vi "HW3_2017_WMA.vi"() -> ()   [LabVIEW 2017]
panel:
  in  "OK Button 2":bool
  in  "Path":path
  in  "min":dbl
  in  "hour":dbl
  in  "OK Button":bool
  out "Boolean":bool
  in  "SET ALARM":bool
  out "ALARMING TIME":string
  out "DATE":string
  in  "reinstate":bool
  in  "sec":dbl
  in  "min":dbl
  in  "hour":dbl
  in  "reset":bool
  out "sec":dbl(knob) scale=0.0..60.0
  out "min":dbl(knob) scale=0.0..60.0
  out "hour":dbl(knob) scale=0.0..12.0
  in  "stop":bool
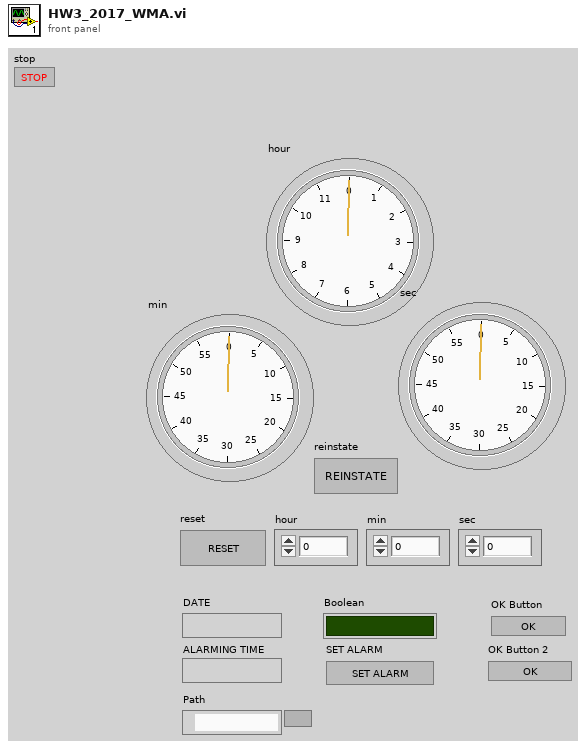
[diagram p1: front panel]
types:
  T1 = typedef "LVDateTimeRec.ctl" = cluster{"fractional second":dbl, "second":i32, "minute":i32, "hour":i32, "day of month":i32, "month":i32, "year":i32, "day of week":i32, "day of year":i32, "DST":i32}
  T2 = typedef "Sound Output Task ID.ctl" = u32
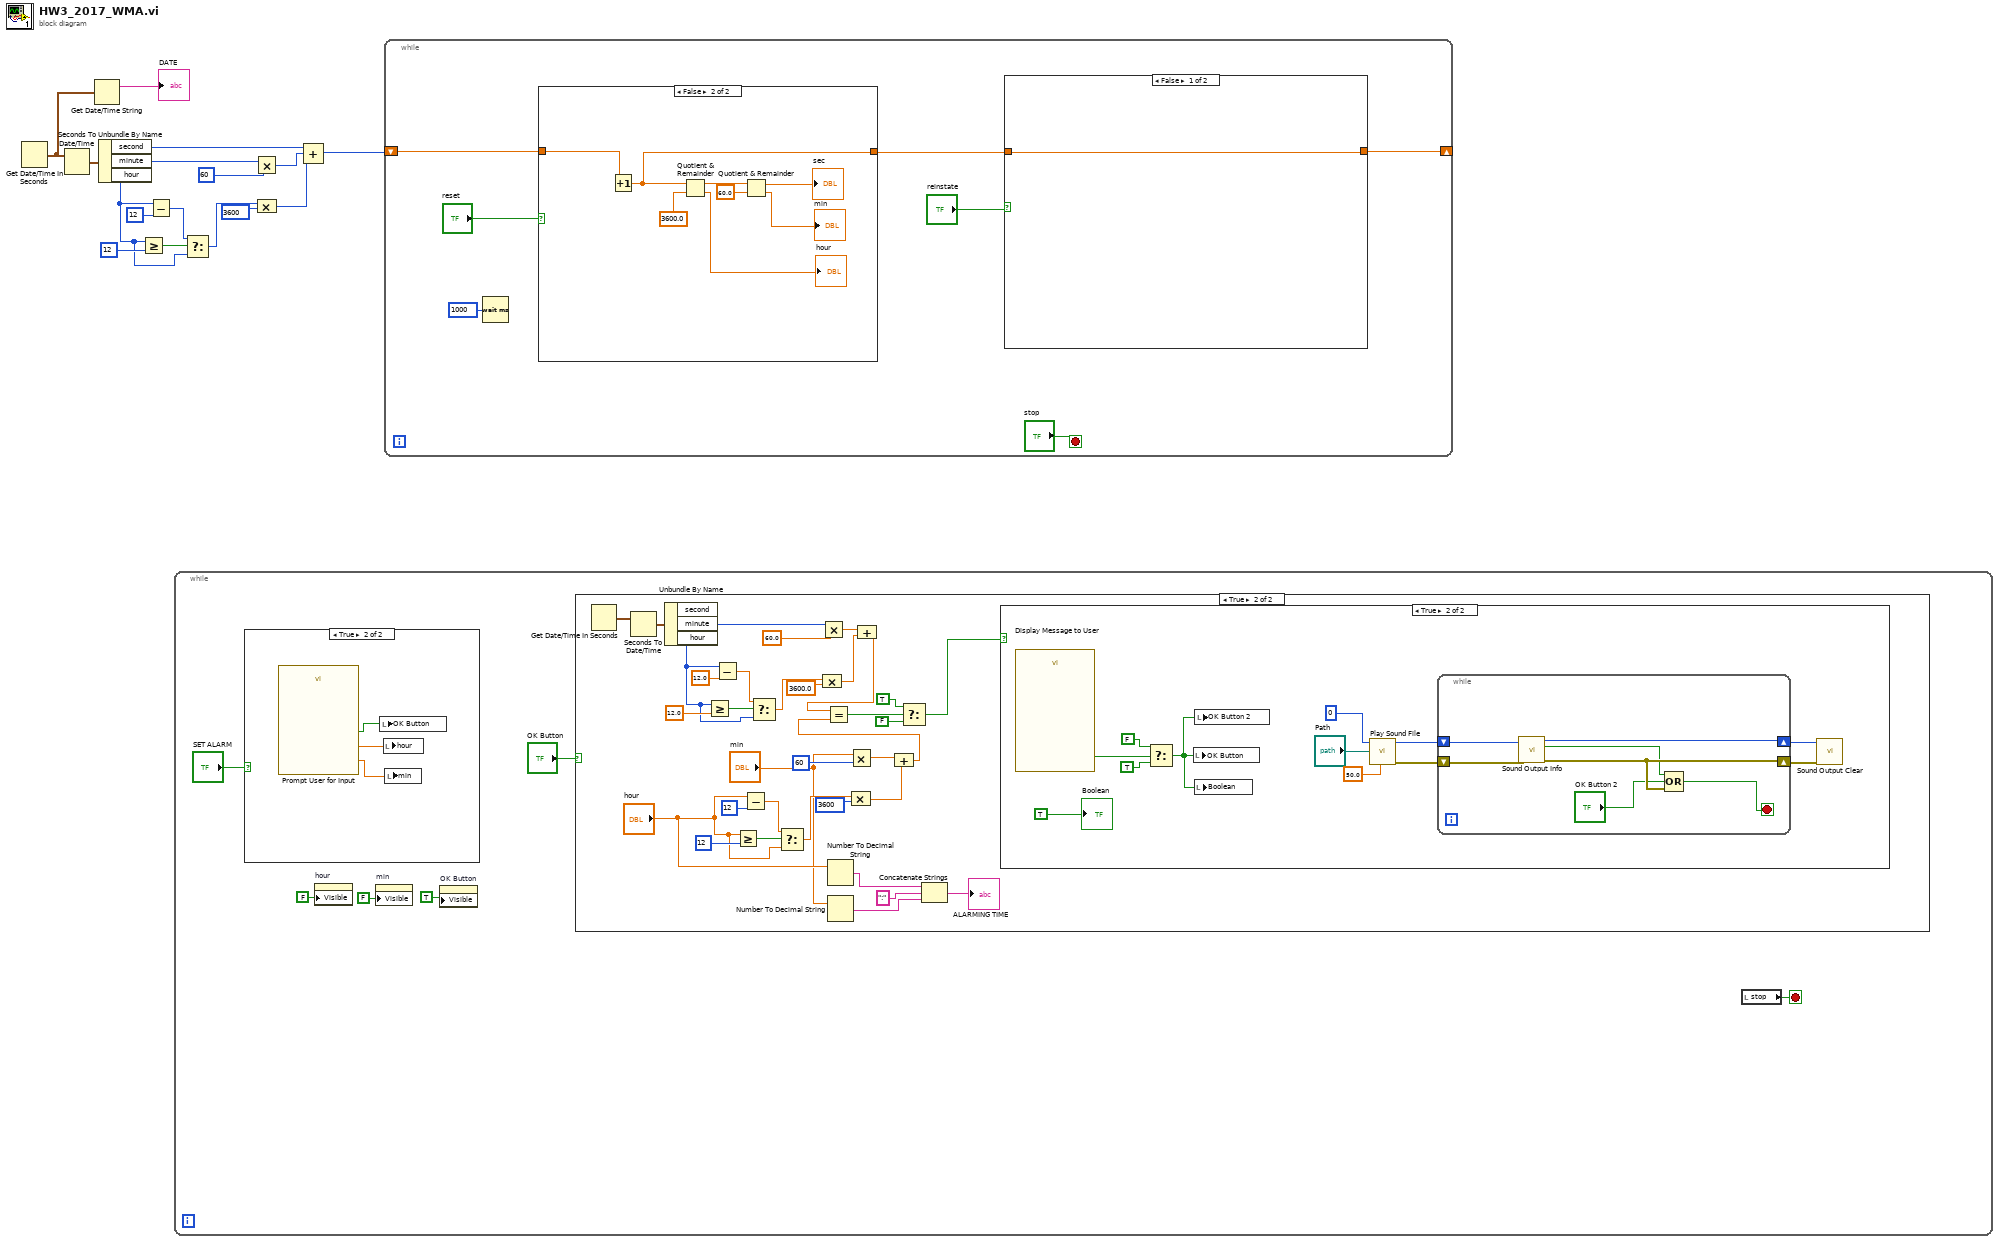
[diagram p0: block diagram]
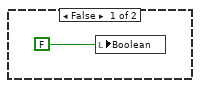
[diagram p3: hidden frame]
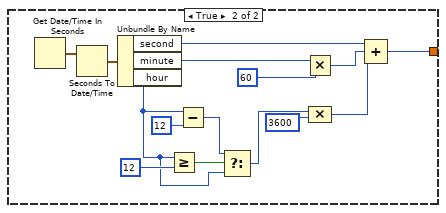
[diagram p5: hidden frame]
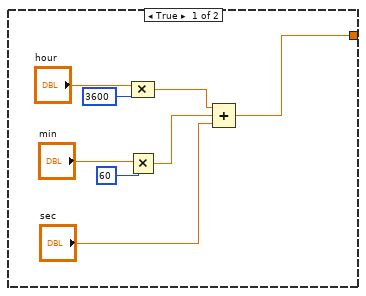
[diagram p6: hidden frame]
diagram:
  n1 = Get Date/Time In Seconds() -> (seconds since 1Jan1904=w5:timestamp)
  n2 = Seconds To Date/Time(time stamp (now)=w5) -> (date time rec=w14:T1)  [unwired: 1 in]
  n3 = Get Date/Time String(seconds (now)=w5) -> (date string=→"DATE":string)  [unwired: 2 in, 1 out]
  n4 = Unbundle By Name(w14) -> ("second"=w12:i32, "minute"=w13:i32, "hour"=w7:i32)
  n5 = Greater Or Equal?(x=w7, y=12) -> (x >= y?=w10:bool)
  n6 = Subtract(x=w7, y=12) -> (x-y=w8:i32)
  n7 = while {
    stop <- w18 stop-if-true
    n8 = case shown="True" "SET ALARM" {
      frame False {
      }
      frame True {
        n9 = call "Prompt User for Input"() -> ("Minute"=w79:dbl, "Hour"=w78:dbl, "OK"=w77:bool)  [unwired: 16 in, 1 out]
        n10 = local write "OK Button"(w77) -> ()
        n11 = local write "hour"(w78) -> ()
        n12 = local write "min"(w79) -> ()
      }
    }
    n13 = property on="hour" class="DigNum (strict)"("Visible"=FALSE) -> ()  [unwired: 2 in, 2 out]
    n14 = property on="min" class="DigNum (strict)"("Visible"=FALSE) -> ()  [unwired: 2 in, 2 out]
    n15 = property on="OK Button" class="Bool (strict)"("Visible"=TRUE) -> ()  [unwired: 2 in, 2 out]
    n16 = case shown="True" "OK Button" {
      frame False {
      }
      frame True {
        n17 = Get Date/Time In Seconds() -> (seconds since 1Jan1904=w26:timestamp)
        n18 = Seconds To Date/Time(time stamp (now)=w26) -> (date time rec=w29:T1)  [unwired: 1 in]
        n19 = Unbundle By Name(w29) -> ("minute"=w30:i32, "hour"=w24:i32)  [unwired: 1 out]
        n20 = Greater Or Equal?(x=w24, y=12.0) -> (x >= y?=w32:bool)
        n21 = Subtract(x=w24, y=12.0) -> (x-y=w34:dbl)
        n22 = Greater Or Equal?(x="hour", y=12) -> (x >= y?=w51:bool)
        n23 = Subtract(x="hour", y=12) -> (x-y=w49:dbl)
        n24 = Select(t=w34, s=w32, f=w24) -> (s? t:f=w35:dbl)
        n25 = Select(t=w49, s=w51, f="hour") -> (s? t:f=w48:dbl)
        n26 = Multiply(x=w30, y=60.0) -> (x*y=w36:dbl)
        n27 = Compound Arithmetic op=MULTIPLY(w35, 3600.0) -> (w37:dbl)
        n28 = Number To Decimal String(number="hour") -> (decimal integer string=w43:string)  [unwired: 1 in]
        n29 = Number To Decimal String(number="min") -> (decimal integer string=w41:string)  [unwired: 1 in]
        n30 = Multiply(x="min", y=60) -> (x*y=w54:dbl)
        n31 = Compound Arithmetic op=MULTIPLY(w48, 3600) -> (w53:dbl)
        n32 = Compound Arithmetic op=ADD(w36, w37) -> (w25:dbl)
        n33 = Compound Arithmetic op=ADD(w54, w53) -> (w47:dbl)
        n34 = Equal?(x=w25, y=w47) -> (x = y?=w46:bool)
        n35 = Select(t=TRUE, s=w46, f=FALSE) -> (s? t:f=w23:bool)
        n36 = Concatenate Strings(w43, ":", w41) -> (→"ALARMING TIME":string)
        n37 = case shown="True" w23 {
          frame False {
            n38 = local write "Boolean"(FALSE ("Boolean")) -> ()
          }
          frame True {
            n39 = call "Display Message to User"() -> ("OK"=w67:bool)  [unwired: 10 in, 1 out]
            n40 = Select(t=FALSE ("Boolean"), s=w67, f=TRUE) -> (s? t:f=w58:bool)
            n41 = local write "OK Button"(w58) -> ()
            n42 = local write "Boolean"(w58) -> ()
            n43 = local write "OK Button 2"(w58) -> ()
            n44 = call <vilib>:"Play Sound File.vi"("timeout (sec)"=50.0, "path"="Path", "device ID"=u32 0) -> ("error out"=w62:errorcluster, "task ID"=w63:T2)  [unwired: 7 in]
            n45 = while {
              shift-right: [w74] -> w61
              shift-left: w63 -> [w76]
              shift-right: [w73] -> w60
              shift-left: w62 -> [w75]
              stop <- w70 stop-if-true
              n46 = call <vilib>:"Sound Output Info.vi"("error in (no error)"=w75, "task ID"=w76) -> ("error out"=w73:errorcluster, "is playing?"=w71:bool, "task ID out"=w74:T2)  [unwired: 6 in, 1 out]
              n47 = Compound Arithmetic op=OR(w71, "OK Button 2", w73) -> (w70:bool)
            }
            n48 = call <vilib>:"Sound Output Clear.vi"("error in (no error)"=w60, "task ID"=w61) -> ()  [unwired: 9 in, 1 out]
            "Boolean" <- TRUE ("Boolean")
          }
        }
      }
    }
    n49 = local read "stop"() -> (w18:bool)
  }
  n50 = Select(t=w8, s=w10, f=w7) -> (s? t:f=w6:i32)
  n51 = Multiply(x=w13, y=60) -> (x*y=w2:i32)
  n52 = Compound Arithmetic op=MULTIPLY(w6, 3600) -> (w1:i32)
  n53 = Compound Arithmetic op=ADD(w12, w2, w1) -> (w4:i32)
  n54 = while {
    shift-right: [w81] -> _
    shift-left: w4 -> [w85]
    stop <- "stop" stop-if-true
    n55 = Wait (ms)(milliseconds to wait=u32 1000) -> ()  [unwired: 1 out]
    n56 = case shown="False" "reset" {
      tunnel: w85 -> [_ w118]
      tunnel: [w103 w111] -> w82
      frame True {
        n57 = Multiply(x="min", y=60) -> (x*y=w105:dbl)
        n58 = Compound Arithmetic op=MULTIPLY("hour", 3600) -> (w106:dbl)
        n59 = Compound Arithmetic op=ADD(w106, w105, "sec") -> (w103:dbl)
      }
      frame False {
        n60 = Increment(x=w118) -> (x+1=w111:dbl)
        n61 = Quotient & Remainder(x=w111, y=3600.0) -> (x-y*floor(x/y)=w116:dbl, floor(x/y)=→"hour":dbl)
        n62 = Quotient & Remainder(x=w116, y=60.0) -> (x-y*floor(x/y)=→"sec":dbl, floor(x/y)=→"min":dbl)
      }
    }
    n63 = case shown="False" "reinstate" {
      tunnel: w82 -> [w87 _]
      tunnel: [w87 w88] -> w81
      frame False {
      }
      frame True {
        n64 = Get Date/Time In Seconds() -> (seconds since 1Jan1904=w99:timestamp)
        n65 = Seconds To Date/Time(time stamp (now)=w99) -> (date time rec=w98:T1)  [unwired: 1 in]
        n66 = Unbundle By Name(w98) -> ("second"=w95:i32, "minute"=w97:i32, "hour"=w90:i32)
        n67 = Greater Or Equal?(x=w90, y=12) -> (x >= y?=w93:bool)
        n68 = Subtract(x=w90, y=12) -> (x-y=w91:i32)
        n69 = Select(t=w91, s=w93, f=w90) -> (s? t:f=w89:i32)
        n70 = Multiply(x=w97, y=60) -> (x*y=w100:i32)
        n71 = Compound Arithmetic op=MULTIPLY(w89, 3600) -> (w96:i32)
        n72 = Compound Arithmetic op=ADD(w95, w100, w96) -> (w88:i32)
      }
    }
  }
